vi "Light VISA Global.vi"() -> ()   [LabVIEW 2025]
panel:
  out "LIGHT VISA resource name out":refnum<visa-resource-name>
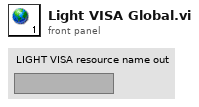
[diagram p1: front panel]
diagram:
